vi "Transition State.vi"(8 "error in (no error)":errorcluster, 10 "Next State":string, 11 "Iteration Actions in":refnum<class "Iteration Actions.lvclass">) -> (0 "error out":errorcluster, 3 "Iteration Actions out":refnum<class "Iteration Actions.lvclass">)   [LabVIEW 2020, in "VolatusSeq.lvlib" / "Iteration Actions.lvclass"]
uses:
  Iteration Actions.lvclass
  Iteration Actions.lvclass/Iteration Actions.ctl
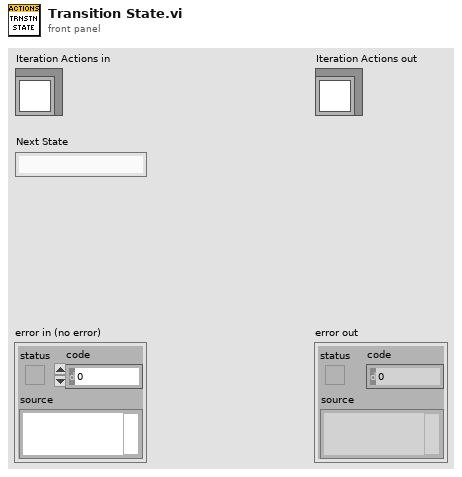
[diagram p1: front panel]
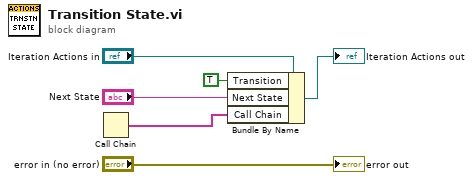
[diagram p0: block diagram]
diagram:
  n1 = Call Chain() -> (call chain=w1:string[])
  n2 = Bundle By Name(cluster="Iteration Actions in", "Transition"=TRUE, "Next State"="Next State", "Call Chain"=w1) -> (→"Iteration Actions out":refnum<class "Iteration Actions.lvclass">)
  "error out" <- "error in (no error)"
